vi "NXT_ Init Tugboat Properties.vi"() -> (0 "Tugboat Properties":T1)   [LabVIEW 2012, in "Tugboat.lvrbt"]
uses:
  Tugboat.lvrbt
  tugProperties_t.ctl
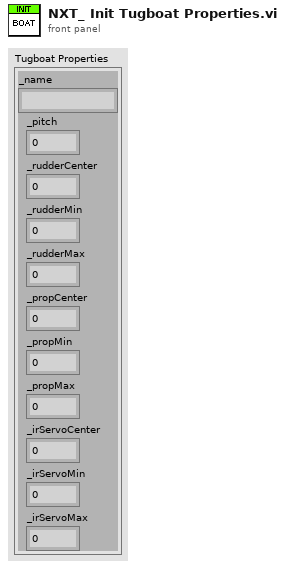
[diagram p1: front panel]
types:
  T1 = typedef "tugProperties_t.ctl" = cluster{"_name":string, "_pitch":u16, "_rudderCenter":u16, "_propCenter":u16, "_irServoCenter":u16, "_rudderMin":u16, "_rudderMax":u16, "_propMin":u16, "_propMax":u16, "_irServoMin":u16, "_irServoMax":u16}
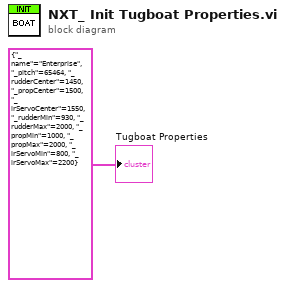
[diagram p0: block diagram]
diagram:
  "Tugboat Properties" <- T1 {"_name"="Enterprise", "_pitch"=65464, "_rudderCenter"=1450, "_propCenter"=1500, "_irServoCenter"=1550, "_rudderMin"=930, "_rudderMax"=2000, "_propMin"=1000, "_propMax"=2000, "_irServoMin"=800, "_irServoMax"=2200} ("Tugboat Properties")
